vi "Resistance to Word.vi"(11 "Resistance":dbl) -> (3 "Resistance Word":u16 format="%016b")   [LabVIEW 2014, in "SLSC configuration Shared.lvlib"]
uses:
  SLSC configuration Shared.lvlib
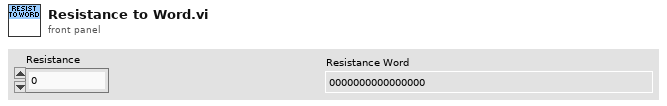
[diagram p1: front panel]
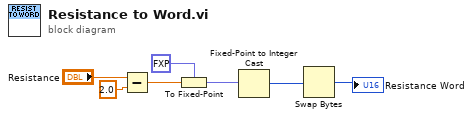
[diagram p0: block diagram]
diagram:
  n1 = Subtract(x="Resistance", y=2.0) -> (x-y=w5:dbl)
  n2 = To Fixed-Point(fixed-point type=fxp<+,16,13> 0.0, number=w5) -> (fixed-point=w3:fxp<+,16,13>)
  n3 = Fixed-Point to Integer Cast(1:w3) -> (0:w2:u16)
  n4 = Swap Bytes(anything=w2) -> (byte swapped=→"Resistance Word":u16)
